vi "BoxEdges-Tri intersection test.vi"(1 "Triangle":T1, 2 "Box":T2={"Face 0"={"V0"=[], "V1"=[], "V2"=[], "V3"=[], "E0"=[], "E1"=[], "E2"=[], "E3"=[], "n^"=[], "Plane"=enum."XY"}, "Face 1"={"V0"=[], "V1"=[], "V2"=[], "V3"=[], "E0"=[], "E1"=[], "E2"=[], "E3"=[], "n^"=[], "Plane"=enum."XY"}, "Face 2"={"V0"=[], "V1"=[], "V2"=[], "V3"=[], "E0"=[], "E1"=[], "E2"=[], "E3"=[], "n^"=[], "Plane"=enum."XY"}, "Face 3"={"V0"=[], "V1"=[], "V2"=[], "V3"=[], "E0"=[], "E1"=[], "E2"=[], "E3"=[], "n^"=[], "Plane"=enum."XY"}, "Face 4"={"V0"=[], "V1"=[], "V2"=[], "V3"=[], "E0"=[], "E1"=[], "E2"=[], "E3"=[], "n^"=[], "Plane"=enum."XY"}, "Face 5"={"V0"=[], "V1"=[], "V2"=[], "V3"=[], "E0"=[], "E1"=[], "E2"=[], "E3"=[], "n^"=[], "Plane"=enum."XY"}, "Level"=-1, "Pmax"=[], "Pmin"=[], "Parent"=-1, "Child 1"=-1, "Child 2"=-1, "Child 3"=-1, "Child 4"=-1, "Child 5"=-1, "Child 6"=-1, "Child 7"=-1, "Child 8"=-1, "Triangles"=[], "is leaf node"=FALSE}) -> (0 "Intersection":bool)   [LabVIEW 2014]
uses:
  Typedefs/TreeNodeBox.ctl
  Typedefs/Quad.ctl
  Typedefs/Quadplane enum.ctl
  Typedefs/Triangle.ctl
  Point-in-Tri test.vi
  Edge-Plane intersection test.vi
  Dot product.vi
panel:
  # "PN 17/01/2015"
  # "Vertices"
  # "Edges"
  # "Unit normal"
  # "Edge unit normals"
  # "Vertices"
  # "Edges"
  # "Unit normal"
  # "Plane ident."
  # "Vertices"
  # "Edges"
  # "Unit normal"
  # "Plane ident."
  # "Vertices"
  # "Edges"
  # "Unit normal"
  # "Plane ident."
  # "Vertices"
  # "Edges"
  # "Unit normal"
  # "Plane ident."
  # "Vertices"
  # "Edges"
  # "Unit normal"
  # "Plane ident."
  # "Vertices"
  # "Edges"
  # "Unit normal"
  # "Plane ident."
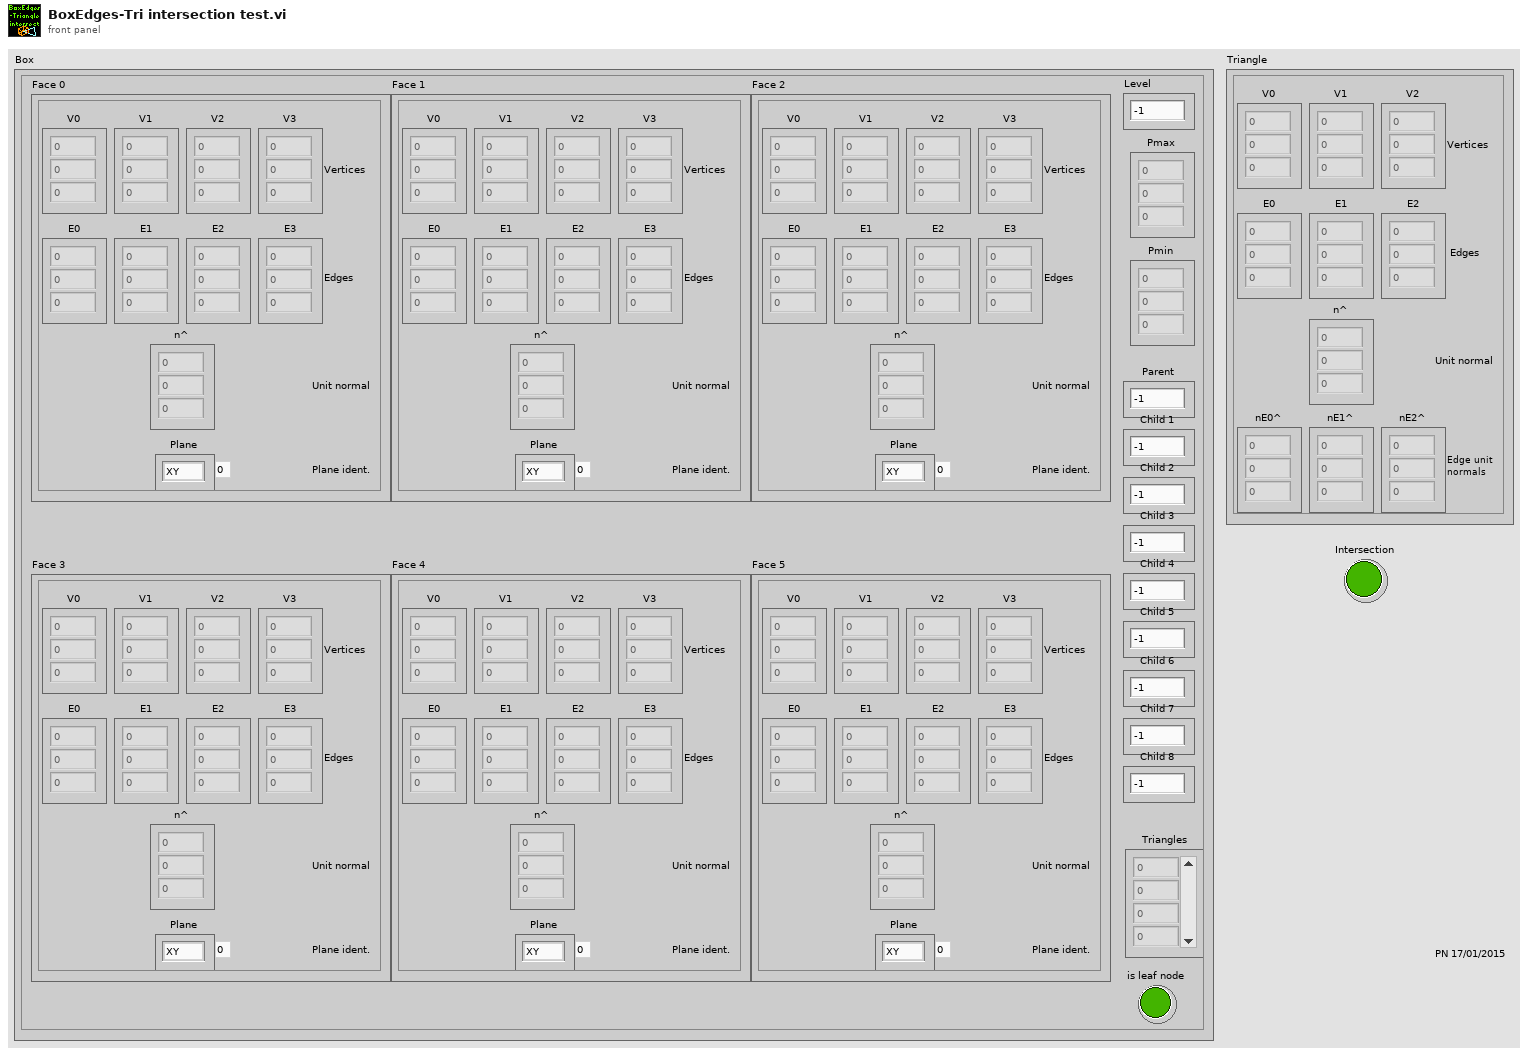
[diagram p1: front panel]
types:
  T1 = typedef "Triangle.ctl" = cluster{"V0":sgl[], "V1":sgl[], "V2":sgl[], "E0":sgl[], "E1":sgl[], "E2":sgl[], "n^":sgl[], "nE0^":sgl[], "nE1^":sgl[], "nE2^":sgl[]}
  T2 = typedef "TreeNodeBox.ctl" = cluster{"Face 0":T3, "Face 1":T3, "Face 2":T3, "Face 3":T3, "Face 4":T3, "Face 5":T3, "Level":i32, "Pmax":sgl[], "Pmin":sgl[], "Parent":i32, "Child 1":i32, "Child 2":i32, "Child 3":i32, "Child 4":i32, "Child 5":i32, "Child 6":i32, "Child 7":i32, "Child 8":i32, "Triangles":i32[], "is leaf node":bool}
  T3 = typedef "Quad.ctl" = cluster{"V0":sgl[], "V1":sgl[], "V2":sgl[], "V3":sgl[], "E0":sgl[], "E1":sgl[], "E2":sgl[], "E3":sgl[], "n^":sgl[], "Plane":T4}
  T4 = typedef "Quadplane enum.ctl" = enum8{"XY", "XZ", "YZ", "-XY", "-XZ", "-YZ"}
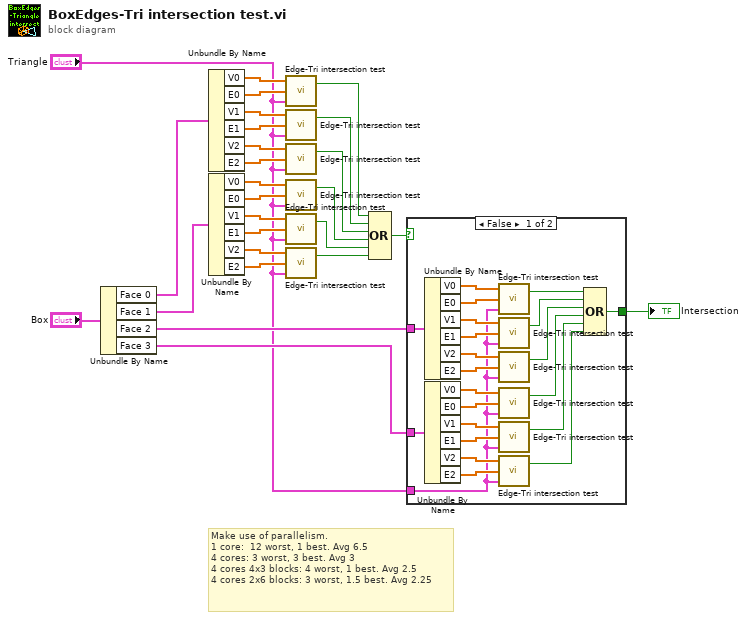
[diagram p0: block diagram]
diagram:
  # "Make use of parallelism.\n1 core:  12 worst, 1 best. Avg 6.5\n4 cores: 3 worst, 3 best. Avg 3\n4 cores 4x3 blocks: 4 worst, 1 best. Avg 2.5\n4 cores 2x6 blocks: 3 worst, 1.5 best. Avg 2.25"
  n1 = Unbundle By Name("Box") -> ("Face 0"=w25:T3, "Face 1"=w12:T3, "Face 2"=w11:T3, "Face 3"=w10:T3)
  n2 = Unbundle By Name(w25) -> ("V0"=w24:sgl[], "E0"=w23:sgl[], "V1"=w22:sgl[], "E1"=w21:sgl[], "V2"=w20:sgl[], "E2"=w19:sgl[])
  n3 = Unbundle By Name(w12) -> ("V0"=w13:sgl[], "E0"=w14:sgl[], "V1"=w15:sgl[], "E1"=w16:sgl[], "V2"=w17:sgl[], "E2"=w18:sgl[])
  n4 = call "Edge-Tri intersection test.vi"("Triangle"="Triangle", "Edge vector (not unit)"=w23, "Edge start point"=w24) -> ("Intersection"=w9:bool)  [unwired: 1 out]
  n5 = call "Edge-Tri intersection test.vi"("Triangle"="Triangle", "Edge vector (not unit)"=w21, "Edge start point"=w22) -> ("Intersection"=w8:bool)  [unwired: 1 out]
  n6 = call "Edge-Tri intersection test.vi"("Triangle"="Triangle", "Edge vector (not unit)"=w19, "Edge start point"=w20) -> ("Intersection"=w7:bool)  [unwired: 1 out]
  n7 = call "Edge-Tri intersection test.vi"("Triangle"="Triangle", "Edge vector (not unit)"=w14, "Edge start point"=w13) -> ("Intersection"=w6:bool)  [unwired: 1 out]
  n8 = call "Edge-Tri intersection test.vi"("Triangle"="Triangle", "Edge vector (not unit)"=w16, "Edge start point"=w15) -> ("Intersection"=w5:bool)  [unwired: 1 out]
  n9 = call "Edge-Tri intersection test.vi"("Triangle"="Triangle", "Edge vector (not unit)"=w18, "Edge start point"=w17) -> ("Intersection"=w4:bool)  [unwired: 1 out]
  n10 = Compound Arithmetic op=OR(w9, w8, w7, w6, w5, w4) -> (w2:bool)
  n11 = case shown="False" w2 {
    selector: w2 -> [_ w49]
    tunnel: w11 -> [w36 _]
    tunnel: w10 -> [w35 _]
    tunnel: "Triangle" -> [w28 _]
    tunnel: [w27 w49] -> w1
    frame False {
      n12 = Unbundle By Name(w36) -> ("V0"=w37:sgl[], "E0"=w38:sgl[], "V1"=w39:sgl[], "E1"=w40:sgl[], "V2"=w41:sgl[], "E2"=w42:sgl[])
      n13 = Unbundle By Name(w35) -> ("V0"=w48:sgl[], "E0"=w47:sgl[], "V1"=w46:sgl[], "E1"=w45:sgl[], "V2"=w44:sgl[], "E2"=w43:sgl[])
      n14 = call "Edge-Tri intersection test.vi"("Triangle"=w28, "Edge vector (not unit)"=w38, "Edge start point"=w37) -> ("Intersection"=w34:bool)  [unwired: 1 out]
      n15 = call "Edge-Tri intersection test.vi"("Triangle"=w28, "Edge vector (not unit)"=w40, "Edge start point"=w39) -> ("Intersection"=w33:bool)  [unwired: 1 out]
      n16 = call "Edge-Tri intersection test.vi"("Triangle"=w28, "Edge vector (not unit)"=w42, "Edge start point"=w41) -> ("Intersection"=w32:bool)  [unwired: 1 out]
      n17 = call "Edge-Tri intersection test.vi"("Triangle"=w28, "Edge vector (not unit)"=w47, "Edge start point"=w48) -> ("Intersection"=w31:bool)  [unwired: 1 out]
      n18 = call "Edge-Tri intersection test.vi"("Triangle"=w28, "Edge vector (not unit)"=w45, "Edge start point"=w46) -> ("Intersection"=w30:bool)  [unwired: 1 out]
      n19 = call "Edge-Tri intersection test.vi"("Triangle"=w28, "Edge vector (not unit)"=w43, "Edge start point"=w44) -> ("Intersection"=w29:bool)  [unwired: 1 out]
      n20 = Compound Arithmetic op=OR(w34, w33, w32, w31, w30, w29) -> (w27:bool)
    }
    frame True {
    }
  }
  "Intersection" <- w1
